vi "Change to Init State.vi"(8 "error in (no error)":errorcluster, 11 "Test UI in":refnum<class "Test UI.lvclass">) -> (0 "error out":errorcluster, 3 "Test UI out":refnum<class "Test UI.lvclass">)   [LabVIEW 2024, in "Test UI.lvlib" / "Test UI.lvclass"]
uses:
  Test UI.lvclass
  Test UI.lvclass/Test UI.ctl
  Test States/Test State Messages/Go to Init Msg/Go to Init Msg.lvclass
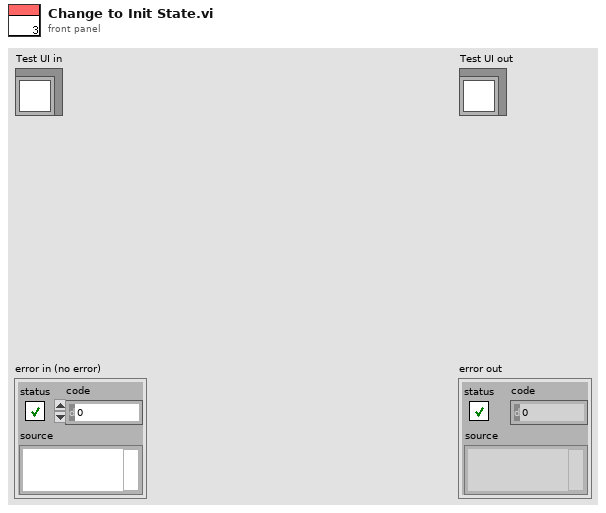
[diagram p1: front panel]
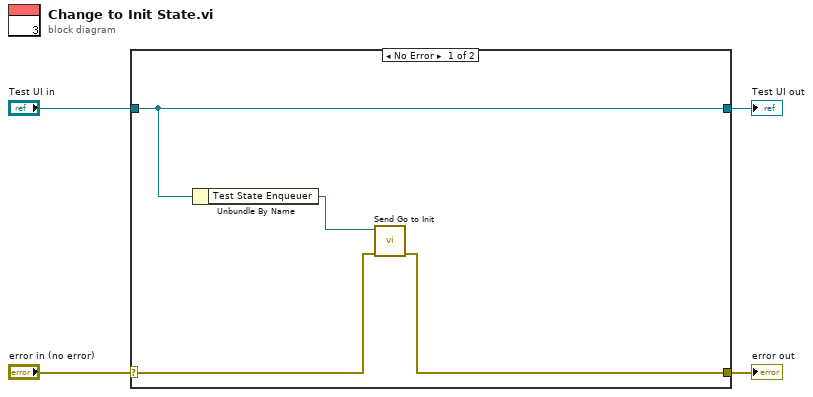
[diagram p0: block diagram]
diagram:
  n1 = case shown="No Error" "error in (no error)" {
    selector: "error in (no error)" -> [w8 w10]
    tunnel: [w6 w10] -> w3
    tunnel: [w7 w9] -> w1
    tunnel: "Test UI in" -> [w7 w9]
    frame No Error {
      n2 = Unbundle By Name(w7) -> ("Test State Enqueuer"=w5:refnum<class "Message Enqueuer.lvclass">)
      n3 = call "Send Go to Init.vi"("error in (no error)"=w8, "Message Enqueuer"=w5) -> ("error out"=w6:errorcluster)  [unwired: 8 in, 1 out]
    }
    frame Error {
    }
  }
  "error out" <- w3
  "Test UI out" <- w1
